vi "FGV_PXI8431rs.vi"(4 "Enum":T1, 5 "End Read on Termination Character?":bool=TRUE, 6 "XON/XOFF Characters":T2={"XON"=enum."DC1", "XOFF"=enum."DC3"}, 7 "Termination Character":u8=10 format="%.0x", 8 "error in (no error)":errorcluster, 9 "Command":string="*IDN?", 10 "Serial Settings":T4={"baud rate"=9600, "data bits"=8, "parity"=enum."None", "stop bits"=10, "flow control"=0} {"flow control" items=["None"=0, "XON/XOFF"=1, "RTS/CTS"=2, "DTR/DSR"=4]; "stop bits" items=["1.0"=10, "1.5"=15, "2.0"=20]; "data bits" min=5 max=8 step=1; "baud rate" items=["75"=75, "110"=110, "134"=134, "150"=150, "300"=300, "600"=600, "1200"=1200, "1800"=1800, "2400"=2400, "4800"=4800, "7200"=7200, "9600"=9600, "14400"=14400, "19200"=19200, "28800"=28800, "38400"=38400, "56000"=56000, "57600"=57600, "115200"=115200, "128000"=128000, "230400"=230400]}, 11 "VISA resource name":refnum<visa-resource-name>="COM1") -> (0 "error out":errorcluster, 1 "Response":string)   [LabVIEW 2017]
uses:
  Serial - Settings.ctl
  controls/Serial - XON-XOFF Characters.ctl
  controls/Serial - ASCII Characters.ctl
  controls/FS_PXI8431rs.ctl
  <vilib>/Instr/_visa.llb/VISA Configure Serial Port (Instr).vi
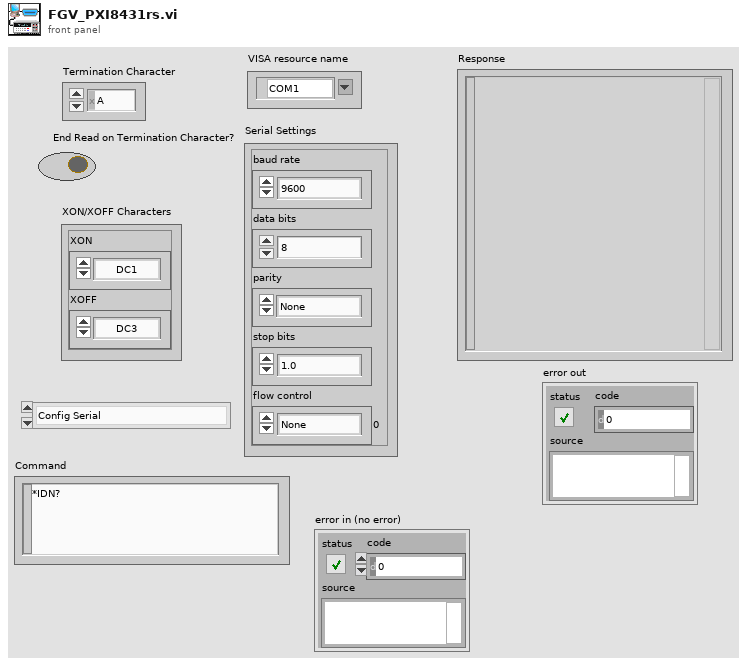
[diagram p1: front panel]
types:
  T1 = typedef "FS_PXI8431rs.ctl" = enum16{"Config Serial", "Xon/Xoff Char", "ASRL TermChar", "Write Command", "Read Data", "Clear Resure"}
  T2 = typedef "Serial - XON-XOFF Characters.ctl" = cluster{"XON":T3, "XOFF":T3}
  T3 = typedef "Serial - ASCII Characters.ctl" = enum16{"NUL", "SOH", "STX", "ETX", "EOT", "ENQ", "ACK", "BEL", "BS", "HT", "LF", "VT", "FF", "CR", "SO", "SI", "DLE", "DC1", "DC2", "DC3", "DC4", "NAK", "SYN", "ETB", "CAN", "EM", "SUB", "ESC", "FS", "GS", "RS", "US", "SP", "!", "\"", "#", "$", "%", "&", "'", "(", ")", "*", "+", ",", "- (-)", ".", "/", "0", "1", "2", "3", "4", "5", "6", "7", "8", "9", ":", ";", "<", "=", ">", "?", "@", "A", "B", "C", "D", "E", "F", "G", "H", "I", "J", "K", "L", "M", "N", "O", "P", "Q", "R", "S", "T", "U", "V", "W", "X", "Y", "Z", "[", "\\", "]", "^", "_", "`", "a", "b", "c", "d", "e", "f", "g", "h", "i", "j", "k", "l", "m", "n", "o", "p", "q", "r", "s", "t", "u", "v", "w", "x", "y", "z", "{", "|", "}", "~"}
  T4 = typedef "Serial - Settings.ctl" = cluster{"baud rate":u32, "data bits":u16, "parity":enum16{"None", "Odd", "Even", "Mark", "Space"}, "stop bits":u16, "flow control":u16}
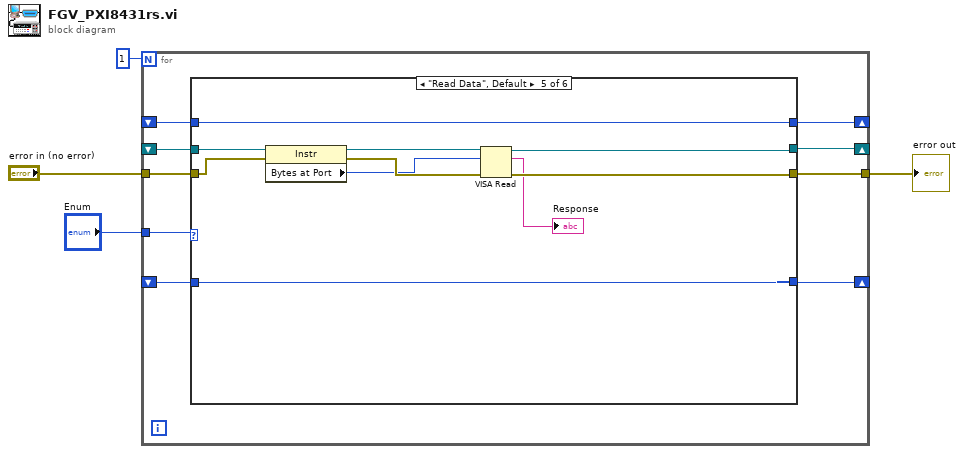
[diagram p0: block diagram]
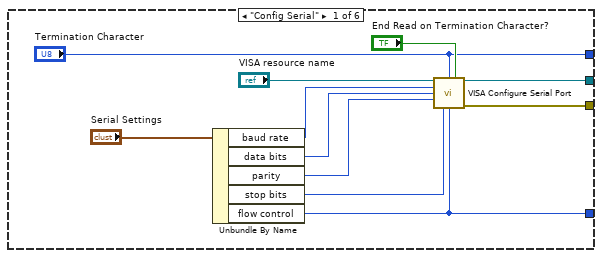
[diagram p2: hidden frame]
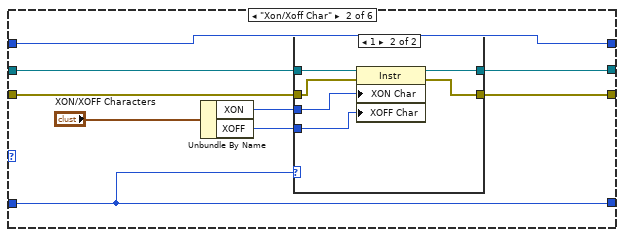
[diagram p3: hidden frame]
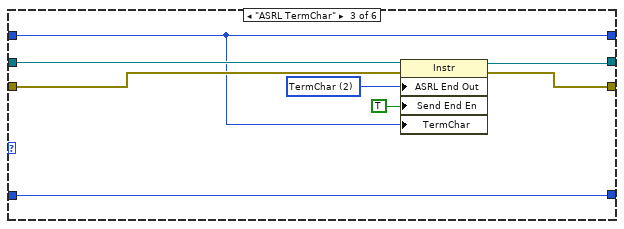
[diagram p5: hidden frame]
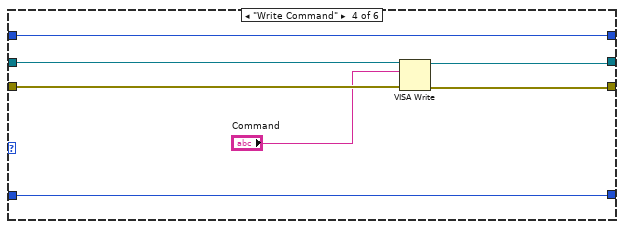
[diagram p6: hidden frame]
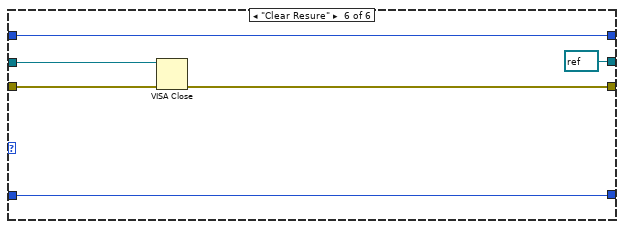
[diagram p7: hidden frame]
diagram:
  n1 = for {
    N: 1 -> [_]
    tunnel: "Enum" -> [w13]
    shift-right: [w11] -> _
    shift-left: _ -> [w10]
    tunnel: [w12] -> w1
    shift-right: [w9] -> _
    shift-left: _ -> [w6]
    shift-right: [w8] -> _
    shift-left: _ -> [w7]
    tunnel: "error in (no error)" -> [w5]
    n2 = case shown="\"Read Data\", Default" w13 {
      tunnel: [w23 w29 w47 w53 w63 w68] -> w12
      tunnel: [w22 w31 w48 w54 w64 refnum<visa-resource-name> refnum ("VISA resource name out")] -> w11
      tunnel: w10 -> [_ w32 w49 w55 w65 w70]
      tunnel: [w16 w33 w42 w50 w62 w71] -> w9
      tunnel: ["Termination Character" w30 w43 w56 w66 w72] -> w8
      tunnel: w7 -> [_ w30 w43 w56 w66 w72]
      tunnel: w6 -> [_ w33 w42 w50 w62 w71]
      tunnel: w5 -> [_ w25 w46 w52 w60 w69]
      frame "Config Serial" {
        n3 = Unbundle By Name("Serial Settings") -> ("baud rate"=w20:u32, "data bits"=w19:u16, "parity"=w18:enum16{"None", "Odd", "Even", "Mark", "Space"}, "stop bits"=w17:u16, "flow control"=w16:u16)
        n4 = call-poly "VISA Configure Serial Port"("VISA resource name"="VISA resource name", "termination char\n(0xA = '\\n' = LF)"="Termination Character", "Enable Termination\nChar (T)"="End Read on Termination Character?", "baud rate (9600)"=w20, "data bits (8)"=w19, "parity (0:none)"=w18, "stop bits (10: 1 bit)"=w17, "flow control (0:none)"=w16) -> ("VISA resource name out"=w22:refnum<visa-resource-name>, "error out"=w23:errorcluster)  [unwired: 6 in]
      }
      frame "Xon/Xoff Char" {
        n5 = Unbundle By Name("XON/XOFF Characters") -> ("XON"=w27:T3, "XOFF"=w26:T3)
        n6 = case shown="1" w33 {
          tunnel: w32 -> [w35 w41]
          tunnel: [w35 w40] -> w31
          tunnel: [w34 w39] -> w29
          tunnel: w27 -> [_ w38]
          tunnel: w26 -> [_ w37]
          tunnel: w25 -> [w34 w36]
          frame 0, Default {
          }
          frame 1 {
            n7 = property class="Instr"(reference=w41, error in=w36, "XON Char"=w38, "XOFF Char"=w37) -> (reference out=w40:refnum<visa-resource-name>, error out=w39:errorcluster)
          }
        }
      }
      frame "ASRL TermChar" {
        w45 = u16 2 items=["None", "Last Bit", "TermChar", "Break"] ("Serial Settings:End Mode for Writes")
        n8 = property class="Instr"(reference=w49, error in=w46, "ASRL End Out"=w45, "Send End En"=TRUE, "TermChar"=w43) -> (reference out=w48:refnum<visa-resource-name>, error out=w47:errorcluster)
      }
      frame "Write Command" {
        n9 = VISA Write(VISA resource name=w55, write buffer="Command", error in (no error)=w52) -> (VISA resource name out=w54:refnum<visa-resource-name>, error out=w53:errorcluster)  [unwired: 1 out]
      }
      frame "Read Data", Default {
        n10 = property class="Instr"(reference=w65, error in=w60) -> (reference out=w61:refnum<visa-resource-name>, error out=w59:errorcluster, "Bytes at Port"=w58:u32)
        n11 = VISA Read(VISA resource name=w61, byte count=w58, error in (no error)=w59) -> (VISA resource name out=w64:refnum<visa-resource-name>, read buffer=→"Response":string, error out=w63:errorcluster)  [unwired: 1 out]
      }
      frame "Clear Resure" {
        n12 = VISA Close(VISA resource name=w70, error in (no error)=w69) -> (error out=w68:errorcluster)
      }
    }
  }
  "error out" <- w1
